vi "Hello.vi"(11 "Name":string) -> (3 "resulting string":string)   [LabVIEW 2021, in "DummyLib.lvlib"]
uses:
  DummyLib.lvlib
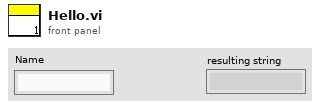
[diagram p1: front panel]
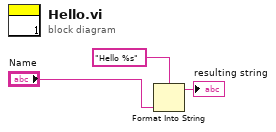
[diagram p0: block diagram]
diagram:
  n1 = Format Into String(format string="Hello %s", "Name") -> (resulting string=→"resulting string":string)  [unwired: 2 in, 1 out]
